vi "Filter Errors.vi"(8 "error in (no error)":errorcluster, 10 "Errors to filter":i32[](array[numeric]), 11 "Error Manager in":refnum<class "Error Manager.lvclass">) -> (0 "error out":errorcluster, 2 "Filters to remove":set{i32}(c389), 3 "Error Manager out":refnum<class "Error Manager.lvclass">)   [LabVIEW 2026, in "TALOS.lvlib" / "Error Manager.lvlib" / "Error Manager.lvclass"]
uses:
  Error Manager.lvclass
  C:/LabVIEW Code/TALOS/talos/Father of all uServices/Father of all uServices/Father of all uServices.lvclass
  Error Manager.lvclass/Error Manager.ctl
  Father of all uServices/Father of all uServices/Father of all uServices.lvclass/Father of all uServices.ctl
  Ancestor/Ancestor/Ancestor.lvclass/Ancestor.ctl
  6bddb594-5bca-43af-9be7-e7ef925c3bc7.vi
  Read Filtered Errors.vi
  Write Filtered Errors.vi
  Support VIs/Substitute Error.vi
  Support VIs/Generate Error.vi
  FGV/Error Memory/Get Error Description.vi
  Support VIs/Get PC name.vi
  Ancestor/Ancestor/Read ID.vi
  Support VIs/Get Class Name.vi
  <vilib>/Utility/error.llb/Clear Errors.vi
  FGV/Error Memory/Error Memory Core.vi
  <vilib>/AdvancedString/Delimited String to 1D String Array.vi
  <vilib>/AdvancedString/Delimited String to 1D String Array (string).vi
  Support VIs/Circus Root Path.vi
  FGV/Error Memory/Error Crt Lvl checker.vi
  FGV/Error Memory/Error Memory Core.vi/40c8088d-b597-4017-91af-faa98e00292e.vi
  FGV/Error Memory/Error Memory Core.vi/d4a3ab98-063c-4e44-b43d-fbdcfe6c2be2.vi
  Support VIs/Global Memory.vi
  <vilib>/Utility/LVClass/Get LV Class Name.vi
  Support VIs/Is in Packed Library.vi
  Support VIs/TALOS Root path.vi
  Support VIs/Read CSV worksheet.vi
  Support VIs/Global Constants.vi
  <vilib>/Utility/error.llb/General Error Handler.vi
  Support VIs/Error Log.vi
  Ancestor/Ancestor/Ancestor.lvclass
  <vilib>/Comparison/Equal/Equal Functor/Equal Functor.lvclass
  Father of all uServices/Father of all uServices/Father of all uServices.lvclass
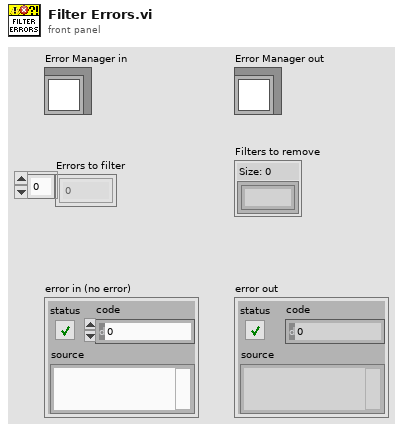
[diagram p1: front panel]
types:
  T1 = typedef "TALOS.lvlib/Error Manager.lvlib/Error Manager.lvclass/Error Info.ctl" = cluster{"error out":errorcluster, "Time Stamp":timestamp, "Machine Name":string, "GUID":string}
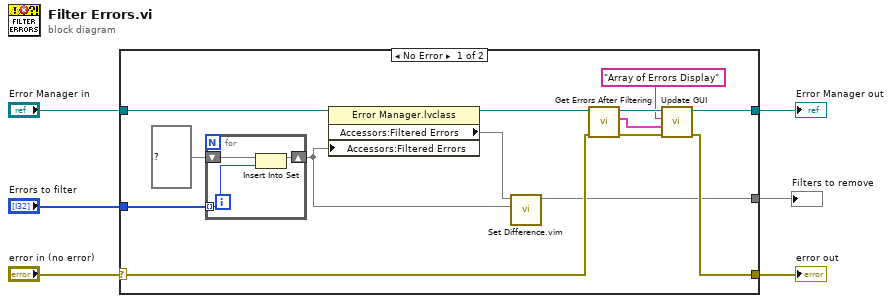
[diagram p0: block diagram]
diagram:
  n1 = case shown="No Error" "error in (no error)" {
    selector: "error in (no error)" -> [w13 w24]
    tunnel: [w19 w25] -> w6
    tunnel: [w18 w24] -> w5
    tunnel: "Errors to filter" -> [w12 _]
    tunnel: "Error Manager in" -> [w11 w25]
    tunnel: [w7 _] -> w1
    frame No Error {
      n2 = for {
        tunnel: w12 -> [w22] mode=indexing
        shift-right: [w21] -> w8
        shift-left: set{i32} {} ("Filtered Errors") -> [w23]
        n3 = Insert Into Set(10:w22, 11:w23) -> (3:w21:set{i32})  [unwired: 1 out]
      }
      n4 = property class="Error Manager.lvclass"(reference=w11, "Accessors:Filtered Errors"=w8) -> (reference out=w10:refnum<class "Error Manager.lvclass">, "Accessors:Filtered Errors"=w9:set{i32})  [unwired: 1 in, 1 out]
      n5 = call "Set Difference.vim"("set 2"=w8, "set 1"=w9) -> ("difference"=w7:set{i32})  [unwired: 9 in]
      n6 = call-dynamic "Get Errors After Filtering.vi"("error in (no error)"=w13, "Error Manager in"=w10) -> ("error out"=w16:errorcluster, "Array of Errors"=w17:T1[], "Error Manager out"=w15:refnum<class "Error Manager.lvclass">)  [unwired: 7 in]
      n7 = call "Update GUI.vi"("error in (no error)"=w16, "Data"=w17, "GUI Item Name"="Array of Errors Display" ("FP Item Name"), "uService Template in"=w15) -> ("error out"=w18:errorcluster, "uService Template out"=w19:refnum<class "Error Manager.lvclass">)  [unwired: 6 in]
    }
    frame Error {
    }
  }
  "Error Manager out" <- w6
  "error out" <- w5
  "Filters to remove" <- w1
